vi "AWGclientHTTP.vi"() -> ()   [LabVIEW 2017]
uses:
  <vilib>/httpClient/POSTBuffer.vi
  <vilib>/httpClient/LabVIEWHTTPClient.lvlib
panel:
  in  "String":string="== RF pulses ==\nshapedPulse 4\nPREP: Cooling\nTime: 6500.0 Step: 0 IQ: 2 Chans: 2 TimingArray: 0\n amp: 200 amp step: 0 channelArray: 111110.54,0,0,0\n amp: 200 amp step: 0 channelArray: 88907.6,0,0,0\nshapedPulse 3\nMW Padding\nTime: 40.0 Step: 0 IQ: 2 Chans: 1 TimingArray: 0\n amp: 0 amp step: 0 channelArray: 0,0,0,0\nshapedPulse 3\nRF Padding\nTime: 40.0 Step: 0 IQ: 1 Chans: 1 TimingArray: 0\n amp: 0 amp step: 0 channelArray: 0,0,0,0\nshapedPulse 3\nMW Padding\nTime: 800.0 Step: 0 IQ: 2 Chans: 1 TimingArray: 0\n amp: 0 amp step: 0 channelArray: 0,0,0,0\nshapedPulse 3\nRF Padding\nTime: 800.0 Step: 0 IQ: 1 Chans: 1 TimingArray: 0\n amp: 0 amp step: 0 channelArray: 0,0,0,0\nshapedPulse 4\nPREP: Cooling\nTime: 6500.0 Step: 0 IQ: 2 Chans: 2 TimingArray: 0\n amp: 200 amp step: 0 channelArray: 111110.54,0,0,0\n amp: 200 amp step: 0 channelArray: 88907.6,0,0,0\nshapedPulse 3\nMW Padding\nTime: 40.0 Step: 0 IQ: 2 Chans: 1 TimingArray: 0\n amp: 0 amp step: 0 channelArray: 0,0,0,0\nshapedPulse 3\nRF Padding\nTime: 40.0 Step: 0 IQ: 1 Chans: 1 TimingArray: 0\n amp: 0 amp step: 0 channelArray: 0,0,0,0\nshapedPulse 3\nFreq scan pluss\nTime: 135.0 Step: 0 IQ: 2 Chans: 1 TimingArray: 0\n amp: 40.0 amp step: 0 channelArray: 111100.54,1,0,0\nshapedPulse 3\nMW Padding\nTime: 800.0 Step: 0 IQ: 2 Chans: 1 TimingArray: 0\n amp: 0 amp step: 0 channelArray: 0,0,0,0\nshapedPulse 3\nRF Padding\nTime: 800.0 Step: 0 IQ: 1 Chans: 1 TimingArray: 0\n amp: 0 amp step: 0 channelArray: 0,0,0,0\nshapedPulse 4\nLine trig set\nTime: 10 Step: 0 IQ: 2 Chans: 2 TimingArray: 0\n amp: 200 amp step: 0 channelArray: 111110.54,0,0,0\n amp: 200 amp step: 0 channelArray: 88907.6,0,0,0\n"
  out "body":string
  out "headers":string
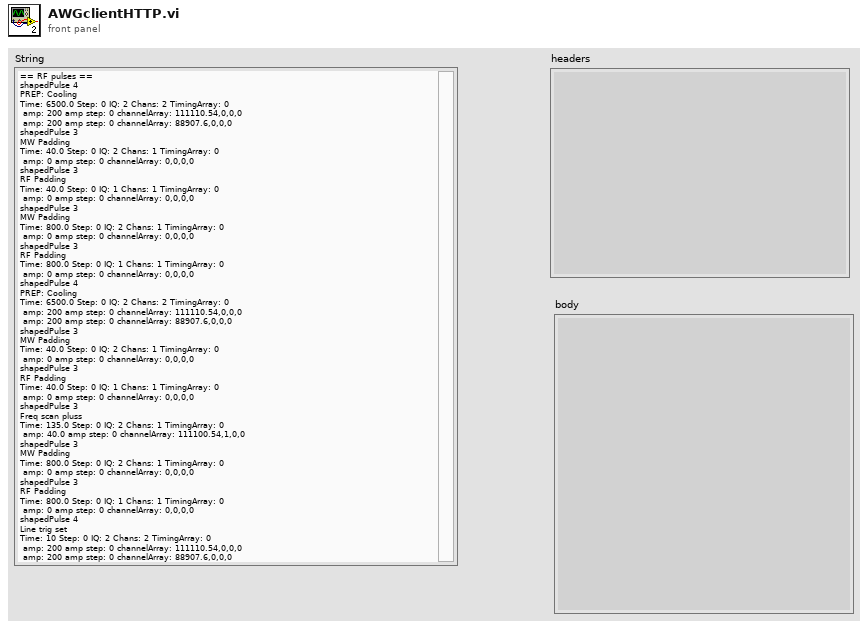
[diagram p1: front panel]
types:
  T1 = typedef "LabVIEWHTTPClient.lvlib/ClientHandle.ctl" = refnum<k1>
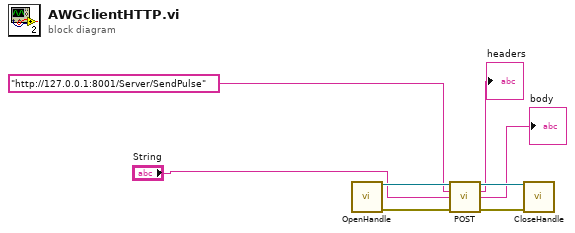
[diagram p0: block diagram]
diagram:
  n1 = call <vilib>:"OpenHandle.vi"() -> ("client handle out"=w8:T1, "error out"=w5:errorcluster)  [unwired: 14 in]
  n2 = call-poly <vilib>:"POST.vi"("client handle"=w8, "url"="http://127.0.0.1:8001/Server/SendPulse", "buffer"="String", "error in (no error)"=w5) -> ("client handle out"=w7:T1, "headers"=→"headers":string, "body"=→"body":string, "error out"=w6:errorcluster)  [unwired: 8 in]
  n3 = call <vilib>:"CloseHandle.vi"("client handle"=w7, "error in (no error)"=w6) -> ()  [unwired: 13 in, 1 out]
